vi "Thev-Compute Equivalent Source.vi"(0 "Px":cdb[][](array[numeric]), 7 "Zx":cdb[][](array[numeric])) -> (4 "Ps":cdb[](array[numeric]), 8 "Zs":cdb[](array[numeric]))   [LabVIEW 2015]
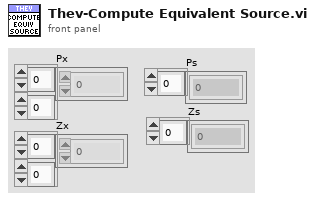
[diagram p1: front panel]
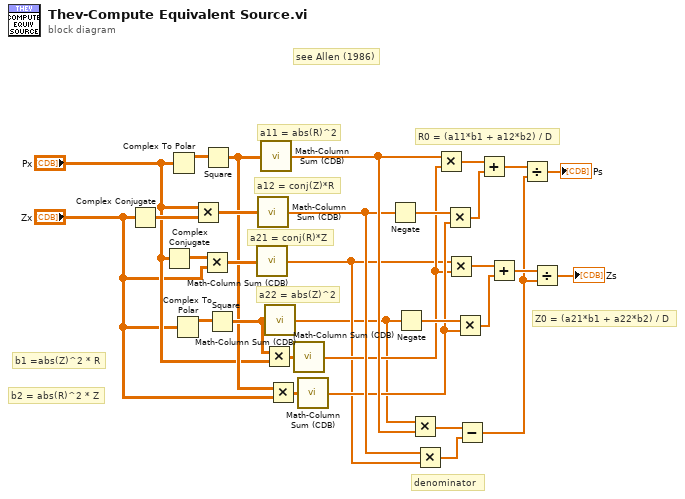
[diagram p0: block diagram]
diagram:
  # "see Allen (1986)"
  # "Z0 = (a21*b1 + a22*b2) / D"
  # "R0 = (a11*b1 + a12*b2) / D"
  # "b2 = abs(R)^2 * Z"
  # "b1 =abs(Z)^2 * R"
  # "denominator"
  # "a22 = abs(Z)^2"
  # "a21 = conj(R)*Z"
  # "a12 = conj(Z)*R"
  # "a11 = abs(R)^2"
  n1 = Complex Conjugate(1:"Zx") -> (0:w30:cdb[][])
  n2 = Complex Conjugate(1:"Px") -> (0:w28:cdb[][])
  n3 = Complex To Polar(r * e^(i*theta)="Px") -> (r=w31:dbl[][])  [unwired: 1 out]
  n4 = Complex To Polar(r * e^(i*theta)="Zx") -> (r=w26:dbl[][])  [unwired: 1 out]
  n5 = Multiply(x="Px", y=w30) -> (x*y=w29:cdb[][])
  n6 = Multiply(x=w28, y="Zx") -> (x*y=w27:cdb[][])
  n7 = Square(x=w31) -> (x^2=w20:dbl[][])
  n8 = Square(x=w26) -> (x^2=w23:dbl[][])
  n9 = call "Math-Column Sum (CDB).vi"("2D Array"=w27) -> ("Column sums"=w7:cdb[])
  n10 = call "Math-Column Sum (CDB).vi"("2D Array"=w29) -> ("Column sums"=w18:cdb[])
  n11 = call "Math-Column Sum (CDB).vi"("2D Array"=w20) -> ("Column sums"=w19:cdb[])
  n12 = Multiply(x=w23, y="Px") -> (x*y=w22:cdb[][])
  n13 = call "Math-Column Sum (CDB).vi"("2D Array"=w23) -> ("Column sums"=w6:cdb[])
  n14 = Multiply(x=w20, y="Zx") -> (x*y=w21:cdb[][])
  n15 = call "Math-Column Sum (CDB).vi"("2D Array"=w22) -> ("Column sums"=w8:cdb[])
  n16 = call "Math-Column Sum (CDB).vi"("2D Array"=w21) -> ("Column sums"=w9:cdb[])
  n17 = Negate(x=w18) -> (-x=w17:cdb[])
  n18 = Negate(x=w6) -> (-x=w13:cdb[])
  n19 = Multiply(x=w6, y=w19) -> (x*y=w25:cdb[])
  n20 = Multiply(x=w18, y=w7) -> (x*y=w24:cdb[])
  n21 = Multiply(x=w19, y=w8) -> (x*y=w16:cdb[])
  n22 = Multiply(x=w17, y=w9) -> (x*y=w14:cdb[])
  n23 = Multiply(x=w7, y=w8) -> (x*y=w12:cdb[])
  n24 = Multiply(x=w13, y=w9) -> (x*y=w10:cdb[])
  n25 = Subtract(x=w25, y=w24) -> (x-y=w5:cdb[])
  n26 = Add(x=w16, y=w14) -> (x+y=w15:cdb[])
  n27 = Add(x=w12, y=w10) -> (x+y=w11:cdb[])
  n28 = Divide(x=w15, y=w5) -> (x/y=→"Ps":cdb[])
  n29 = Divide(x=w11, y=w5) -> (x/y=→"Zs":cdb[])
